vi "DumpToLog.vi"(11 "DataToLog":string[](array[string])) -> ()   [LabVIEW 2017]
uses:
  <vilib>/Utility/sysdir.llb/System Directory Type.ctl
panel:
  out "error out":errorcluster
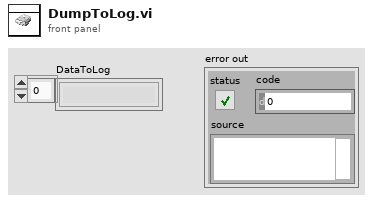
[diagram p1: front panel]
types:
  T1 = enum16{"open", "replace", "create", "open or create", "replace or create", "replace or create with confirmation"}
  T2 = typedef "System Directory Type.ctl" = i32
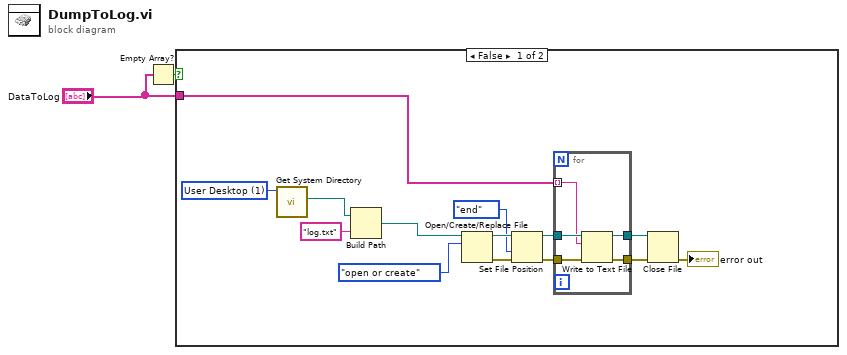
[diagram p0: block diagram]
diagram:
  n1 = Empty Array?(array="DataToLog") -> (empty?=w1:bool)
  n2 = case shown="False" w1 {
    tunnel: "DataToLog" -> [w7 _]
    frame False {
      w3 = T2 1 items=["User Home"=0, "User Desktop"=1, "User Documents"=2, "User Application Data"=3, "User Preferences"=4, "User Temporary"=5, "Public Documents"=6, "Public Application Data"=7, "Public Preferences"=8, "Public Cache"=13, "System Core Libraries"=9, "System Installed Libraries"=10, "Application Files"=11, "Boot Volume Root"=12] ("system directory type")
      n3 = call <vilib>:"Get System Directory.vi"("system directory type"=w3) -> ("system directory"=w6:path)  [unwired: 10 in]
      n4 = Build Path(base path=w6, name or relative path="log.txt") -> (appended path=w4:path)
      n5 = Open/Create/Replace File(file path (use dialog)=w4, operation (0:open)=T1."open or create") -> (refnum out=w15:refnum<file>, error out=w14:errorcluster)  [unwired: 4 in, 1 out]
      n6 = Set File Position(refnum=w15, from (0:start)=enum16{"start", "end", "current"}."end", error in=w14) -> (refnum out=w13:refnum<file>, error out=w12:errorcluster)  [unwired: 1 in]
      n7 = for {
        tunnel: w13 -> [w21]
        tunnel: w12 -> [w20]
        tunnel: w7 -> [w19] mode=indexing
        tunnel: [w18] -> w10
        tunnel: [w17] -> w9
        n8 = Write to Text File(file (use dialog)=w21, text=w19, error in=w20) -> (refnum out=w18:refnum<file>, error out=w17:errorcluster)  [unwired: 1 in, 1 out]
      }
      n9 = Close File(refnum=w10, error in=w9) -> (error out=→"error out":errorcluster)  [unwired: 1 out]
    }
    frame True {
    }
  }
